vi "SetFileSeq.vi"(1 "Filename":string, 2 "Sequence":i32 min=0) -> (0 "Filename Out":string)   [LabVIEW 2014]
uses:
  globals/AzCamGlobals.vi
panel:
  out "match substring":string
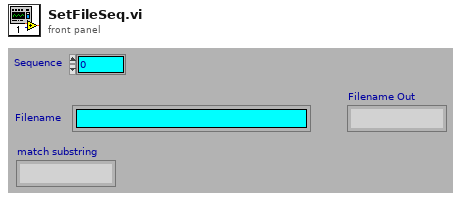
[diagram p1: front panel]
types:
  T1 = enum16{"FITS", "Extended FITS", "Binary", "TIFF", "JPEG", "GIF", "Thumbnail"}
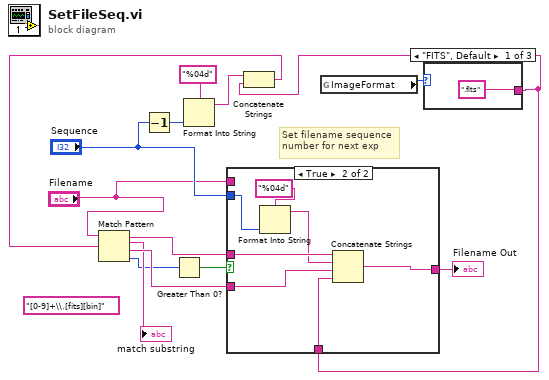
[diagram p0: block diagram]
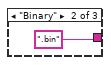
[diagram p2: hidden frame]
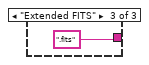
[diagram p3: hidden frame]
diagram:
  (unwired) "[0-9]+\\.[fits][bin]" ("regular expression")
  # "Set filename sequence\nnumber for next exp"
  n1 = Decrement(x="Sequence") -> (x-1=w6:i32)
  n2 = Format Into String(format string="%04d", w6) -> (resulting string=w5:string)  [unwired: 2 in, 1 out]
  n3 = global read "AzCamGlobals.vi" "ImageFormat"() -> (w4:T1)
  n4 = case shown="\"FITS\", Default" w4 {
    tunnel: [".fits" ".bin" ".fits"] -> w2
    frame "FITS", Default {
    }
    frame "Binary" {
    }
    frame "Extended FITS" {
    }
  }
  n5 = Concatenate Strings(w5, w2) -> (w3:string)
  n6 = Match Pattern(string="Filename", regular expression=w3) -> (before substring=w14:string, match substring=→"match substring":string, after substring=w13:string, offset past match=w9:i32)  [unwired: 1 in]
  n7 = Greater Than 0?(x=w9) -> (x > 0?=w10:bool)
  n8 = case shown="True" w10 {
    tunnel: w14 -> [_ w25]
    tunnel: w13 -> [_ w21]
    tunnel: [w18 w19] -> w11
    tunnel: "Filename" -> [w18 _]
    tunnel: "Sequence" -> [_ w23]
    tunnel: w2 -> [_ w20]
    frame False {
    }
    frame True {
      n9 = Format Into String(format string="%04d", w23) -> (resulting string=w22:string)  [unwired: 2 in, 1 out]
      n10 = Concatenate Strings(w25, w22, w21, w20) -> (w19:string)
    }
  }
  "Filename Out" <- w11
